vi "mod_SymbolCntToBitCnt.vi"(2 "Bits/ Symbol":i32=2, 3 "Tx Sequence (Symbols)":T1) -> (0 "M (numeric)":i32, 1 "Tx Sequence (Bits)":T2)   [LabVIEW 2020, in "niDMT.lvlib"]
uses:
  <vilib>/addons/Modulation/niDMT.lvlib
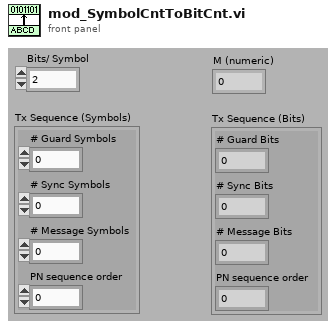
[diagram p1: front panel]
types:
  T1 = cluster{"# Guard Symbols":i32, "# Sync Symbols":i32, "# Message Symbols":i32, "PN sequence order":i32}
  T2 = cluster{"# Guard Bits":i32, "# Sync Bits":i32, "# Message Bits":i32, "PN sequence order":i32}
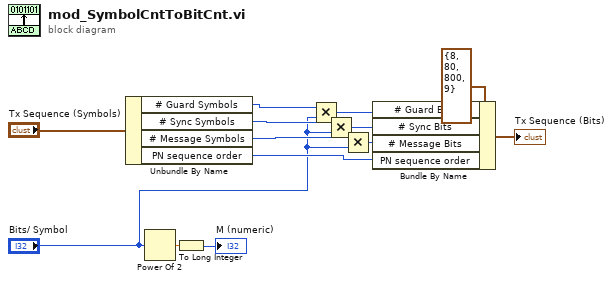
[diagram p0: block diagram]
diagram:
  n1 = Unbundle By Name("Tx Sequence (Symbols)") -> ("# Guard Symbols"=w9:i32, "# Sync Symbols"=w8:i32, "# Message Symbols"=w7:i32, "PN sequence order"=w10:i32)
  n2 = Power Of 2(x="Bits/ Symbol") -> (2^x=w12:dbl)
  n3 = To Long Integer(number=w12) -> (32bit integer=→"M (numeric)":i32)
  n4 = Multiply(x=w9, y="Bits/ Symbol") -> (x*y=w6:i32)
  n5 = Multiply(x=w8, y="Bits/ Symbol") -> (x*y=w4:i32)
  n6 = Multiply(x=w7, y="Bits/ Symbol") -> (x*y=w5:i32)
  n7 = Bundle By Name(cluster=T2 {"# Guard Bits"=8, "# Sync Bits"=80, "# Message Bits"=800, "PN sequence order"=9} ("Message"), "# Guard Bits"=w6, "# Sync Bits"=w4, "# Message Bits"=w5, "PN sequence order"=w10) -> (→"Tx Sequence (Bits)":T2)
